vi "Read Response.vi"(8 "error in":errorcluster, 11 "Newport in":refnum<class "Newport.lvclass">) -> (0 "error out":errorcluster, 2 "Success?":bool, 3 "Newport out":refnum<class "Newport.lvclass">)   [LabVIEW 2018, in "Newport.lvlib" / "Newport.lvclass"]
uses:
  Newport.lvclass
  Parent/Axis.lvclass
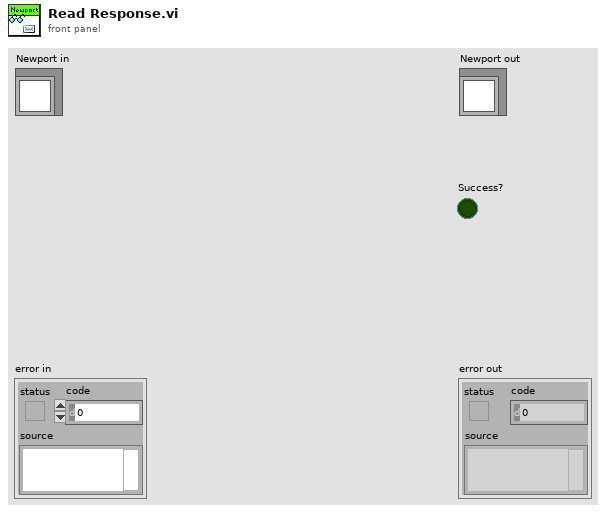
[diagram p1: front panel]
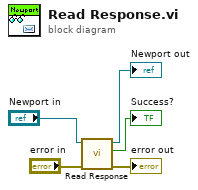
[diagram p0: block diagram]
diagram:
  n1 = call-parent "Read Response.vi"("error in"="error in", "Axis in"="Newport in") -> ("error out"=→"error out":errorcluster, "Success?"=→"Success?":bool, "Axis out"=→"Newport out":refnum<class "Newport.lvclass">)  [unwired: 7 in]
